vi "Rotate3Darray.vi"(11 "ArIn":dbl[][][](array[numeric])) -> (3 "ArOut":dbl[][][](array[numeric]))   [LabVIEW 2014]
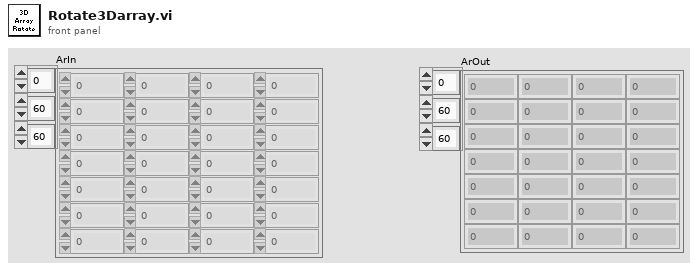
[diagram p1: front panel]
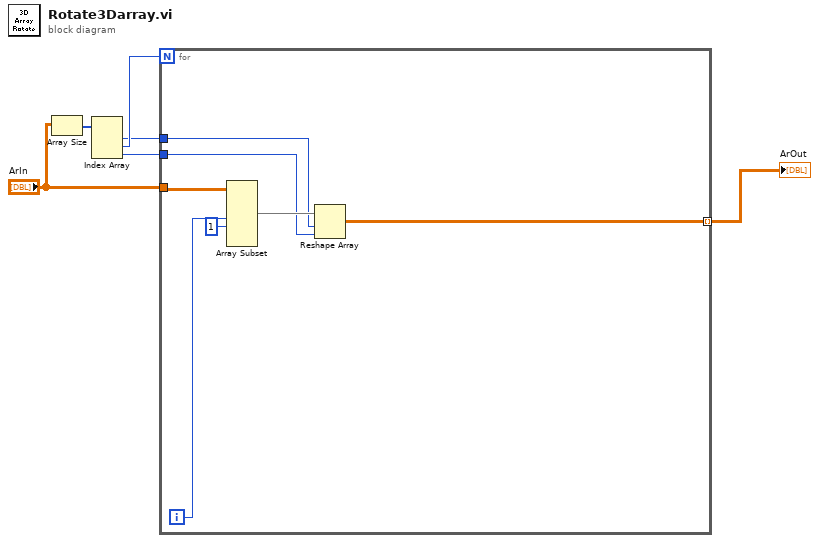
[diagram p0: block diagram]
diagram:
  n1 = Array Size(array="ArIn") -> (size(s)=w6:i32[])
  n2 = Index Array(array=w6) -> (element #1=w3:i32, element #2=w5:i32, element #3=w2:i32)  [unwired: 3 in]
  n3 = for {
    N: w5 -> [_]
    tunnel: "ArIn" -> [w13]
    tunnel: w3 -> [w9]
    tunnel: w2 -> [w8]
    tunnel: [w7] -> w1 mode=indexing
    i -> [w12]
    n4 = Array Subset(array=w13, index (dim 1)=w12, length (dim 1)=1 ("length")) -> (w10:dbl[][][])  [unwired: 4 in]
    n5 = Reshape Array(w10, w9, w8) -> (w7:dbl[][])
  }
  "ArOut" <- w1
